vi "Dynamic Form.vi"(8 "error in (no error)":errorcluster, 9 "FORM outfile":path=path "C:/Users/Murmann-Group/Documents/LabVIEW Data/NI-RRAM-Test-Setup/formout.csv") -> (0 "error out":errorcluster, 1 "final current (A)":dbl, 2 "final resistance (ohm)":dbl format="%#_6p", 3 "final read voltage (V)":dbl, 4 "formed?":bool, 5 "BL voltage (V)":dbl, 7 "WL voltage (V)":dbl)   [LabVIEW 2019]
uses:
  Globals.vi
  <vilib>/Utility/file.llb/Write Delimited Spreadsheet (DBL).vi
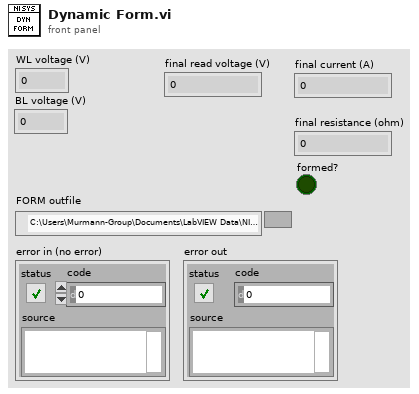
[diagram p1: front panel]
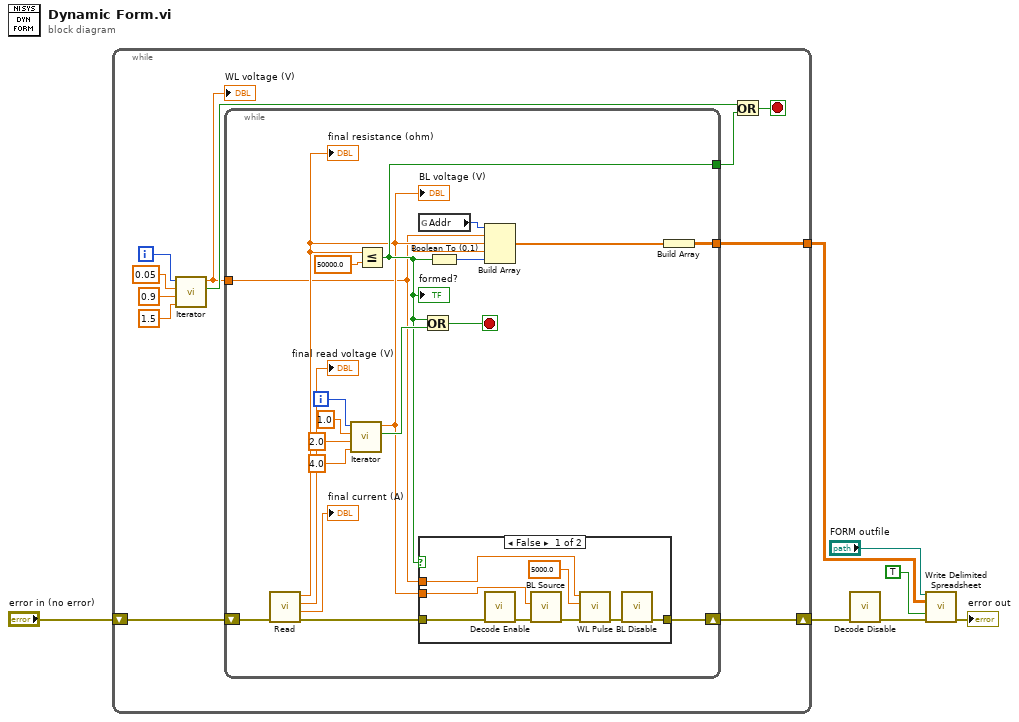
[diagram p0: block diagram]
diagram:
  n1 = while {
    shift-right: [w14] -> w1
    shift-left: "error in (no error)" -> [w12]
    tunnel: [w8] -> w7
    i -> [w15]
    stop <- w16 stop-if-true
    n2 = call "Iterator.vi"("Final Value"=1.5 ("y"), "Initial Value"=0.9 ("y"), "Step"=0.05 ("x"), "i"=w15) -> ("End Loop"=w13:bool, "Current Value"=w9:dbl)  [unwired: 6 in]
    "WL voltage (V)" <- w9
    n3 = while {
      shift-right: [w25] -> w14
      shift-left: w12 -> [w37]
      tunnel: [w28] -> w10
      tunnel: w9 -> [w20]
      tunnel: [w26] -> w8
      i -> [w36]
      stop <- w38 stop-if-true
      n4 = call "Read.vi"("error in (no error)"=w37) -> ("error out"=w19:errorcluster, "current (A)"=→"final current (A)":dbl, "read voltage (V)"=→"final read voltage (V)":dbl, "resistance (ohm)"=w23:dbl)  [unwired: 7 in]
      "final resistance (ohm)" <- w23
      n5 = call "Iterator.vi"("Final Value"=4.0 ("y"), "Initial Value"=2.0 ("y"), "Step"=1.0 ("x"), "i"=w36) -> ("End Loop"=w32:bool, "Current Value"=w27:dbl)  [unwired: 6 in]
      "BL voltage (V)" <- w27
      n6 = Less Or Equal?(x=w23, y=50000.0 ("target resistance (ohm)")) -> (x <= y?=w28:bool)
      "formed?" <- w28
      n7 = global read "Globals.vi" "Addr"() -> (w24:u16)
      n8 = case shown="False" w28 {
        tunnel: [w42 w47] -> w25
        tunnel: w19 -> [w41 w47]
        tunnel: w27 -> [w46 _]
        tunnel: w20 -> [w45 _]
        frame False {
          n9 = call "Decode Enable.vi"("error in (no error)"=w41) -> ("error out"=w40:errorcluster)  [unwired: 10 in]
          n10 = call "BL Source.vi"("error in (no error)"=w40, "voltage level (V)"=w46) -> ("error out"=w44:errorcluster)  [unwired: 9 in]
          n11 = call "WL Pulse.vi"("error in (no error)"=w44, "Sample Rate"=5000.0, "VWL (V)"=w45) -> ("error out"=w43:errorcluster)  [unwired: 8 in]
          n12 = call "BL Disable.vi"("error in (no error)"=w43) -> ("error out"=w42:errorcluster)  [unwired: 10 in]
        }
        frame True {
        }
      }
      n13 = Or(x=w28, y=w32) -> (x .or. y?=w38:bool)
      n14 = Boolean To (0,1)(Boolean=w28) -> (0, 1=w30:i16)
      n15 = Build Array(w24, w20, w27, w23, w30) -> (w29:dbl[])
      n16 = Build Array(w29) -> (w26:dbl[][])
    }
    n17 = Or(x=w13, y=w10) -> (x .or. y?=w16:bool)
  }
  n18 = call "Decode Disable.vi"("error in (no error)"=w1) -> ("error out"=w3:errorcluster)  [unwired: 10 in]
  n19 = call-poly <vilib>:"Write Delimited Spreadsheet.vi"("file path (dialog if empty)"="FORM outfile", "2D data"=w7, "append to file? (new file:F)"=TRUE, "error in (no error)"=w3) -> ("error out"=→"error out":errorcluster)  [unwired: 10 in, 1 out]
